vi "Get Routing and Faulting Custom Device.vi"(8 "error in (no error)":errorcluster, 11 "RAF Custom Device in":refnum<k24>) -> (0 "error out":errorcluster, 2 "Settings":T1, 3 "RAF Custom Device out":refnum<k24>)   [LabVIEW 2017, in "Switch Scripting.lvlib"]
uses:
  Switch Scripting.lvlib
  Shared/Routing and Faulting Custom Device Settings.ctl
  NationalInstruments.VeriStand.SystemDefinitionAPI
  Shared/Switch Shared.lvlib
  <vilib>/NI VeriStand/Custom Device API/Custom Device API.lvlib
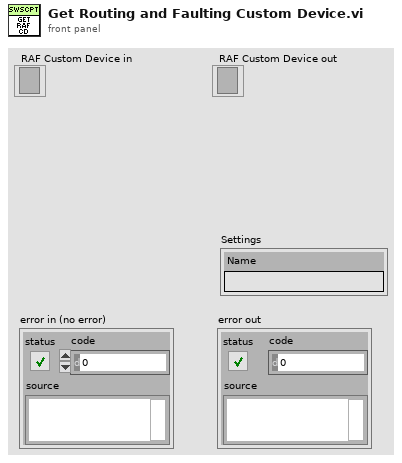
[diagram p1: front panel]
types:
  T1 = typedef "Switch Shared.lvlib/Routing and Faulting Custom Device Settings.ctl" = cluster{"Name":string}
  T2 = typedef "Custom Device API.lvlib/Custom Device Item Info.ctl" = cluster{"Name":string, "Is Channel":bool, "GUID":string, "Is Waveform":bool}
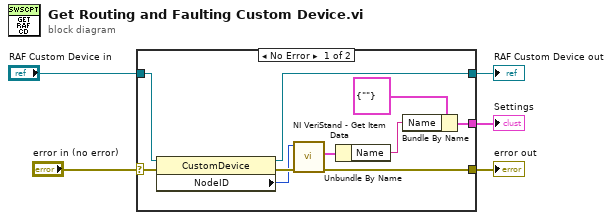
[diagram p0: block diagram]
diagram:
  n1 = case shown="No Error" "error in (no error)" {
    selector: "error in (no error)" -> [w14 w17]
    tunnel: [w6 w17] -> w5
    tunnel: [w15 w16] -> w4
    tunnel: "RAF Custom Device in" -> [w13 w16]
    tunnel: [w12 _] -> w1
    frame No Error {
      n2 = property class="CustomDevice"(reference=w13, error in=w14) -> (reference out=w15:refnum<k24>, error out=w10:errorcluster, "NodeID"=w9:u64)
      n3 = call <vilib>:"NI VeriStand - Get Item Data.vi"("error in (no error)"=w10, "Item Ref in"=w9) -> ("error out"=w6:errorcluster, "Item Info"=w8:T2)  [unwired: 6 in, 2 out]
      n4 = Unbundle By Name(w8) -> ("Name"=w7:string)
      n5 = Bundle By Name(cluster=T1 {"Name"=""} ("Settings"), "Name"=w7) -> (w12:T1)
    }
    frame Error {
    }
  }
  "Settings" <- w1
  "error out" <- w5
  "RAF Custom Device out" <- w4
